vi "ProvetechRBS.vi"(8 "error in (no error)":errorcluster) -> (0 "error out":errorcluster)   [LabVIEW 2020]
uses:
  <vilib>/AKKA/PROVEtech-RBS/TypDefs/RBS Signal.ctl
  <vilib>/AKKA/PROVEtech-RBS/SubVIs/Read (Signals Single-point).vi
  <vilib>/AKKA/PROVEtech-RBS/PROVEtechRBS.lvlib
panel:
  out "size(s) 2":i32
  out "size(s)":i32
  out "RX signals":cluster{"names":string[], "values":dbl[]}
  out "TX signals":cluster{"names":string[], "values":dbl[]}
  out "RBS signal list":T1[](array[typedef])
  out "values":dbl[](array[numeric])
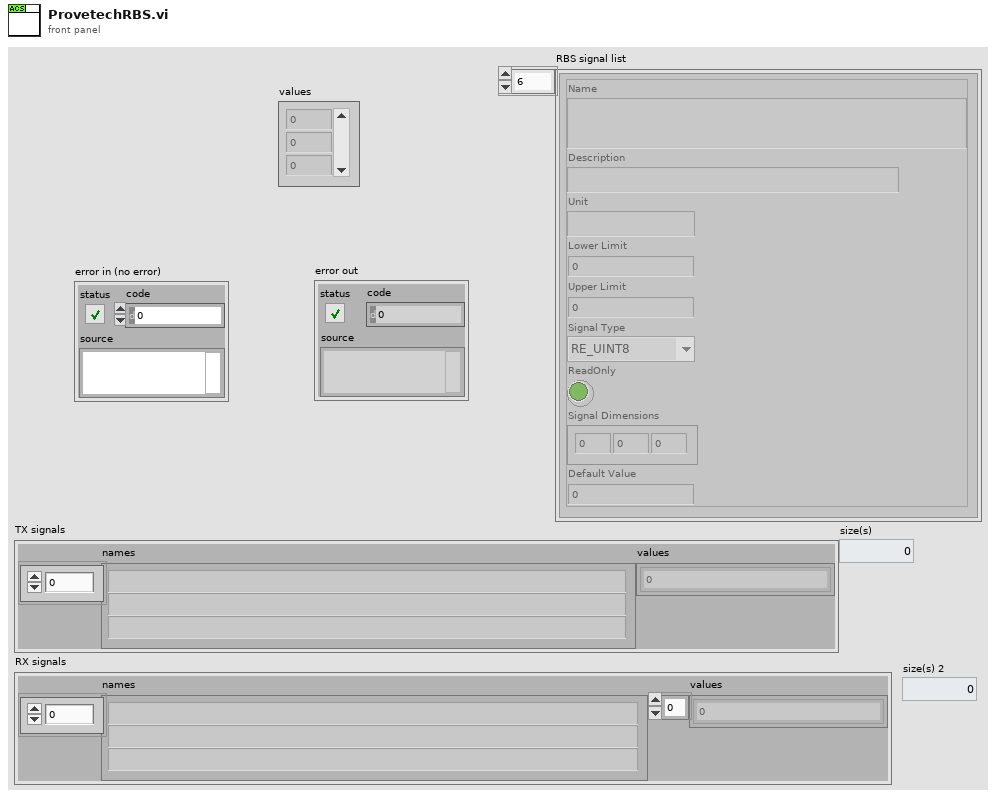
[diagram p1: front panel]
types:
  T1 = typedef "PROVEtechRBS.lvlib/RBS Signal.ctl" = cluster{"Name":string, "Description":string, "Unit":string, "Lower Limit":dbl, "Upper Limit":dbl, "Signal Type":enum32{"RE_UINT8", "RE_INT8", "RE_UINT16", "RE_INT16", "RE_UINT32", "RE_INT32", "RE_UINT64", "RE_INT64", "RE_FLOAT32", "RE_FLOAT64"}, "ReadOnly":bool, "Signal Dimensions":i32[], "Default Value":dbl}
  T2 = typedef "PROVEtechRBS.lvlib/RBS Session.ctl" = cluster{"core":T3, "core VI reference":refnum<vi>}
  T3 = typedef "PROVEtechRBS.lvlib/RBS Core Data.ctl" = cluster{"RBS config file":path, "RBSVeristand path":path, "TX signals":cluster{"names":string[], "values":dbl[]}, "RX signals":cluster{"names":string[], "values":dbl[]}, "TX_enable signals":cluster{"names":string[], "indices":i32[]}, "core comm":cluster{"TX":refnum<data-value>, "RX":refnum<data-value>, "status":refnum<data-value>}}
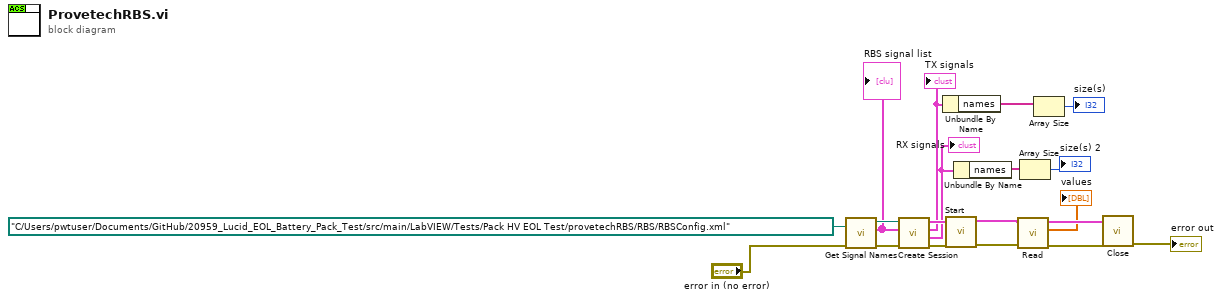
[diagram p0: block diagram]
diagram:
  n1 = call <vilib>:"Get Signal Names.vi"("error in (no error)"="error in (no error)", "RBS config file in"=path "C:/Users/pwtuser/Documents/GitHub/20959_Lucid_EOL_Battery_Pack_Test/src/main/LabVIEW/Tests/Pack HV EOL Test/provetechRBS/RBS/RBSConfig.xml") -> ("error out"=w14:errorcluster, "RBS signal list"=w17:T1[], "RBS config file out"=w18:path)  [unwired: 7 in]
  "RBS signal list" <- w17
  n2 = call <vilib>:"Create Session.vi"("error in (no error)"=w14, "RBS signal list"=w17, "RBS Config File"=w18) -> ("error out"=w13:errorcluster, "RX signals"=w5:cluster{"names":string[], "values":dbl[]}, "TX signals"=w6:cluster{"names":string[], "values":dbl[]}, "RBS session out"=w16:T2)  [unwired: 5 in]
  "TX signals" <- w6
  "RX signals" <- w5
  n3 = Unbundle By Name(w6) -> ("names"=w4:string[])
  n4 = call <vilib>:"Start.vi"("error in (no error)"=w13, "RBS session in"=w16) -> ("error out"=w11:errorcluster, "RBS session out"=w12:T2)  [unwired: 8 in]
  n5 = Unbundle By Name(w5) -> ("names"=w2:string[])
  n6 = call-poly <vilib>:"Read.vi"("error in (no error)"=w11, "RBS session in"=w12) -> ("error out"=w8:errorcluster, "values"=→"values":dbl[], "RBS session out"=w10:T2)  [unwired: 7 in]
  n7 = Array Size(array=w2) -> (size(s)=→"size(s) 2":i32)
  n8 = Array Size(array=w4) -> (size(s)=→"size(s)":i32)
  n9 = call <vilib>:"Close.vi"("error in (no error)"=w8, "RBS session in"=w10) -> ("error out"=→"error out":errorcluster)  [unwired: 9 in]
